vi "SetAxisLabels.vi"(11 "WaveformGraph in":refnum<vi>) -> (0 "error out":errorcluster, 1 "Bounds":T1, 3 "Position":T2)   [LabVIEW 2022 SP3]
uses:
  <vilib>/Utility/miscctls.llb/LVPositionTypeDef.ctl
  <vilib>/Utility/miscctls.llb/LVBoundsTypeDef.ctl
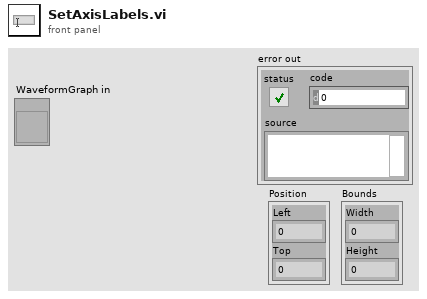
[diagram p1: front panel]
types:
  T1 = typedef "LVBoundsTypeDef.ctl" = cluster{"Width":u32, "Height":u32}
  T2 = typedef "LVPositionTypeDef.ctl" = cluster{"Left":i32, "Top":i32}
  T3 = typedef "LVRectTypeDef.ctl" = cluster{"Left":i16, "Top":i16, "Right":i16, "Bottom":i16}
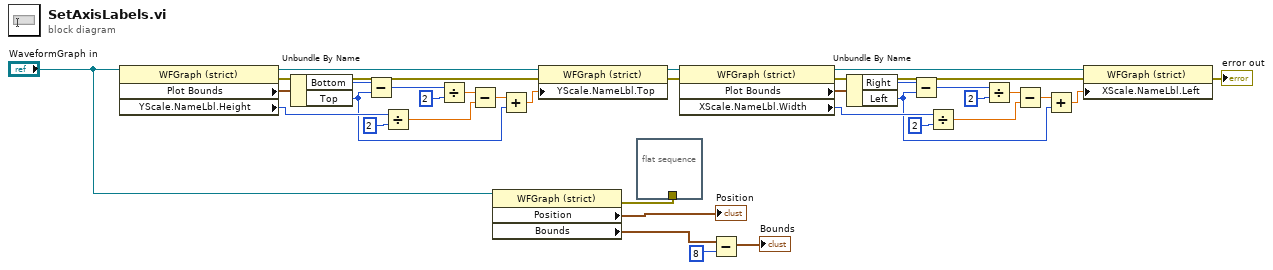
[diagram p0: block diagram]
diagram:
  n1 = property class="WFGraph (strict)"(reference="WaveformGraph in") -> (reference out=w33:refnum<vi>, error out=w9:errorcluster, "Plot Bounds"=w14:T3, "YScale.NameLbl.Height"=w35:u32)  [unwired: 1 in]
  n2 = Unbundle By Name(w14) -> ("Bottom"=w17:i16, "Top"=w16:i16)
  n3 = Subtract(x=w17, y=w16) -> (x-y=w15:i16)
  n4 = Divide(x=w35, y=u32 2) -> (x/y=w13:dbl)
  n5 = Divide(x=w15, y=u32 2) -> (x/y=w18:dbl)
  n6 = Subtract(x=w18, y=w13) -> (x-y=w20:dbl)
  n7 = property on="Property Node" class="WFGraph (strict)"(reference="WaveformGraph in") -> (error out=w1:errorcluster, "Position"=→"Position":T2, "Bounds"=w3:T1)  [unwired: 1 in, 1 out]
  n8 = Add(x=w20, y=w16) -> (x+y=w12:dbl)
  n9 = property class="WFGraph (strict)"(reference=w33, error in=w9, "YScale.NameLbl.Top"=w12) -> (reference out=w28:refnum<vi>, error out=w8:errorcluster)
  n10 = flat-sequence {
    tunnel: w1 -> [_]
    frame #0 {
    }
  }
  n11 = property class="WFGraph (strict)"(reference=w28, error in=w8) -> (reference out=w32:refnum<vi>, error out=w7:errorcluster, "Plot Bounds"=w11:T3, "XScale.NameLbl.Width"=w30:u32)
  n12 = Subtract(x=w3, y=8) -> (x-y=→"Bounds":T1)
  n13 = Unbundle By Name(w11) -> ("Right"=w23:i16, "Left"=w22:i16)
  n14 = Subtract(x=w23, y=w22) -> (x-y=w21:i16)
  n15 = Divide(x=w30, y=u32 2) -> (x/y=w29:dbl)
  n16 = Divide(x=w21, y=u32 2) -> (x/y=w24:dbl)
  n17 = Subtract(x=w24, y=w29) -> (x-y=w27:dbl)
  n18 = Add(x=w27, y=w22) -> (x+y=w26:dbl)
  n19 = property class="WFGraph (strict)"(reference=w32, error in=w7, "XScale.NameLbl.Left"=w26) -> (error out=→"error out":errorcluster)  [unwired: 1 out]
